vi "STA_LTA.vi"(8 "error in (no error)":errorcluster, 10 "waveform in":waveform(sgl)) -> (0 "error out":errorcluster, 1 "valid":bool, 2 "value":dbl)   [LabVIEW 2017]
uses:
  <vilib>/Analysis/baseanly.llb/Mean (DBL).vi
  <vilib>/Analysis/NI_AALBase.lvlib
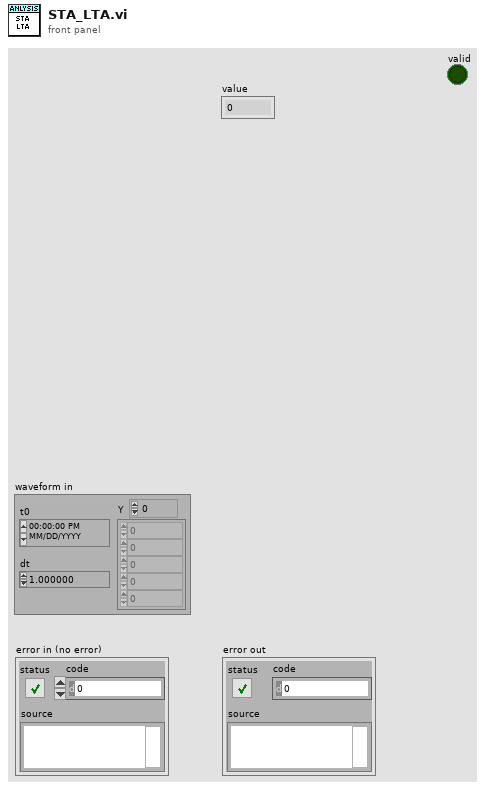
[diagram p1: front panel]
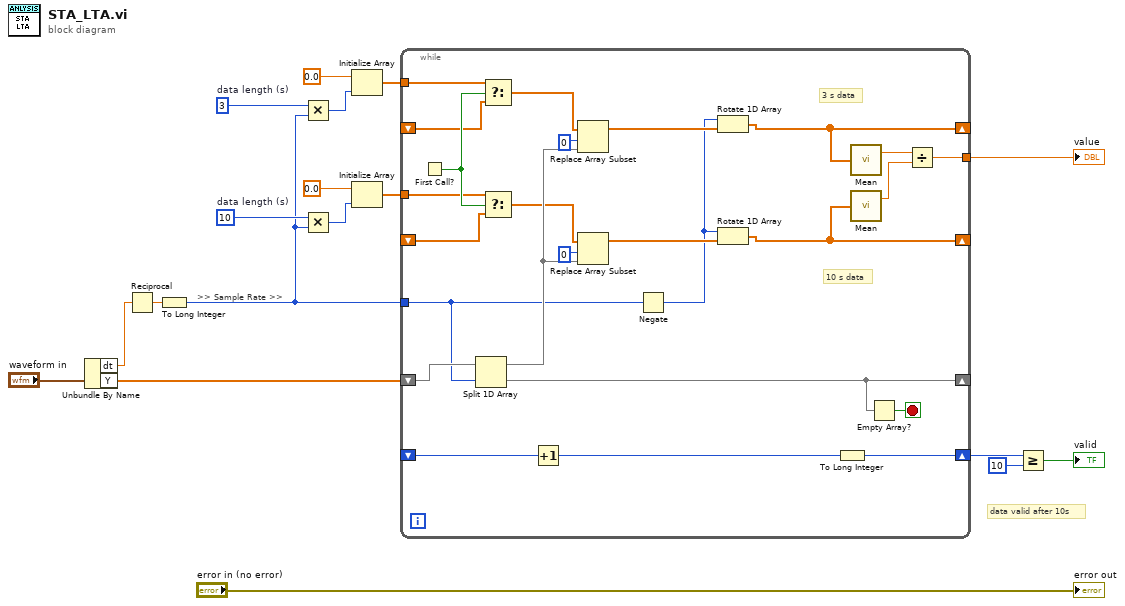
[diagram p0: block diagram]
diagram:
  w13 = 3  # data length (s)
  w16 = 10  # data length (s)
  # "data valid after 10s"
  # ">> Sample Rate >>"
  n1 = Unbundle By Name("waveform in") -> ("dt"=w9:dbl, "Y"=w6:sgl[])
  n2 = Reciprocal(x=w9) -> (1/x=w8:dbl)
  n3 = To Long Integer(number=w8) -> (32bit integer=w7:i32)
  n4 = Multiply(x=w13, y=w7) -> (x*y=w15:i32)
  n5 = Multiply(x=w16, y=w7) -> (x*y=w17:i32)
  n6 = Initialize Array(0.0, w15) -> (w2:dbl[])
  n7 = Initialize Array(0.0, w17) -> (w1:dbl[])
  n8 = while {
    shift-right: [w40] -> _
    shift-left: w6 -> [w43]
    tunnel: w7 -> [w27]
    shift-right: [w34] -> _
    shift-left: _ -> [w20]
    shift-right: [w35] -> _
    shift-left: _ -> [w23]
    tunnel: [w31] -> w10
    shift-right: [w26] -> w5
    shift-left: _ -> [w29]
    tunnel: w2 -> [w24]
    tunnel: w1 -> [w21]
    stop <- w30 stop-if-true
    # "10 s data"
    # "3 s data"
    n9 = First Call?() -> (First Call?: T/F=w25:bool)
    n10 = Split 1D Array(array=w43, index=w27) -> (first subarray=w36:sgl[], second subarray=w40:sgl[])
    n11 = Select(t=w24, s=w25, f=w23) -> (s? t:f=w22:dbl[])
    n12 = Select(t=w21, s=w25, f=w20) -> (s? t:f=w19:dbl[])
    n13 = Increment(x=w29) -> (x+1=w28:i32)
    n14 = Replace Array Subset "Replace Array Subset"(array=w22, new element=w36, index=0) -> (w39:dbl[])
    n15 = Replace Array Subset "Replace Array Subset"(array=w19, new element=w36, index=0) -> (w41:dbl[])
    n16 = Negate(x=w27) -> (-x=w37:i32)
    n17 = Rotate 1D Array(1:w39, 2:w37) -> (0:w35:dbl[])
    n18 = Rotate 1D Array(1:w41, 2:w37) -> (0:w34:dbl[])
    n19 = To Long Integer(number=w28) -> (32bit integer=w26:i32)
    n20 = call-poly <vilib>:"Mean.vi"("X"=w35) -> ("mean"=w33:dbl)  [unwired: 1 out]
    n21 = call-poly <vilib>:"Mean.vi"("X"=w34) -> ("mean"=w32:dbl)  [unwired: 1 out]
    n22 = Empty Array?(array=w40) -> (empty?=w30:bool)
    n23 = Divide(x=w33, y=w32) -> (x/y=w31:dbl)
  }
  "value" <- w10
  n24 = Greater Or Equal?(x=w5, y=10) -> (x >= y?=→"valid":bool)
  "error out" <- "error in (no error)"
